vi "Dictionary New__ogtk.vi"(8 "error in (no error)":errorcluster, 10 "Data in":T2) -> (0 "error out":errorcluster, 3 "Object RefNum":T1)   [LabVIEW 2014]
doc: "Initializes the GOOP object"
uses:
  <userlib>/_OpenG.lib/dictionary/dictionary.llb/Dictionary Data__ogtk.ctl
  <userlib>/_OpenG.lib/dictionary/dictionary.llb/Dictionary Object RefNum__ogtk.ctl
  <userlib>/_OpenG.lib/dictionary/dictionary.llb/Dictionary Object RefNum - Enum__ogtk.ctl
panel:
  # "OpenGOOP New.vi\n\nInitializes the GOOP object\n\nPlease visit http://www.OpenG.org to learn about the\nOpen Source LabVIEW software movement.\n\nNOTICE -- YOU MUST LEAVE THIS NOTICE IN PLACE.  PER THE TERMS OF THE LICENSE BELOW, YOU MAY SUBLICENSE THIS SOFTWARE \nIN ANY WAY THAT DOES NOT CONFLICT WITH THIS LICENSE.\n\n### BSD License (http://www.opensource.org/licenses/bsd-license.php) Begin ###\n \nCopyright (c) 2003, Jim Kring <jim@jimkring.com>\n\nAll rights reserved.\n\nRedistribution and use in source and binary forms, with or without modification, are permitted provided that the following conditions are met:\n\n    * Redistributions of source code must retain the above copyright notice, this list of conditions and the following disclaimer.\n    * Redistributions in binary form must reproduce the above copyright notice, this list of conditions and the following disclaimer in the \n       documentation and/or other materials provided with the distribution.\n    * Neither the name of SciWare, James Kring, Inc., nor the names of its contributors may be used to endorse or promote products derived \n       from this software without specific prior written permission.\n\nTHIS SOFTWARE IS PROVIDED BY THE COPYRIGHT HOLDERS AND CONTRIBUTORS \"AS IS\" AND ANY EXPRESS OR IMPLIED WARRANTIES, \nINCLUDING, BUT NOT LIMITED TO, THE IMPLIED WARRANTIES OF MERCHANTABILITY AND FITNESS FOR A PARTICULAR PURPOSE ARE \nDISCLAIMED. IN NO EVENT SHALL THE COPYRIGHT OWNER OR CONTRIBUTORS BE LIABLE FOR ANY DIRECT, INDIRECT, INCIDENTAL,\n SPECIAL, EXEMPLARY, OR CONSEQUENTIAL DAMAGES (INCLUDING, BUT NOT LIMITED TO, PROCUREMENT OF SUBSTITUTE GOODS OR \nSERVICES; LOSS OF USE, DATA, OR PROFITS; OR BUSINESS INTERRUPTION) HOWEVER CAUSED AND ON ANY THEORY OF LIABILITY, \nWHETHER IN CONTRACT, STRICT LIABILITY, OR TORT (INCLUDING NEGLIGENCE OR OTHERWISE) ARISING IN ANY WAY OUT OF THE USE \nOF THIS SOFTWARE, EVEN IF ADVISED OF THE POSSIBILITY OF SUCH DAMAGE.\n\n### BSD License End ###"
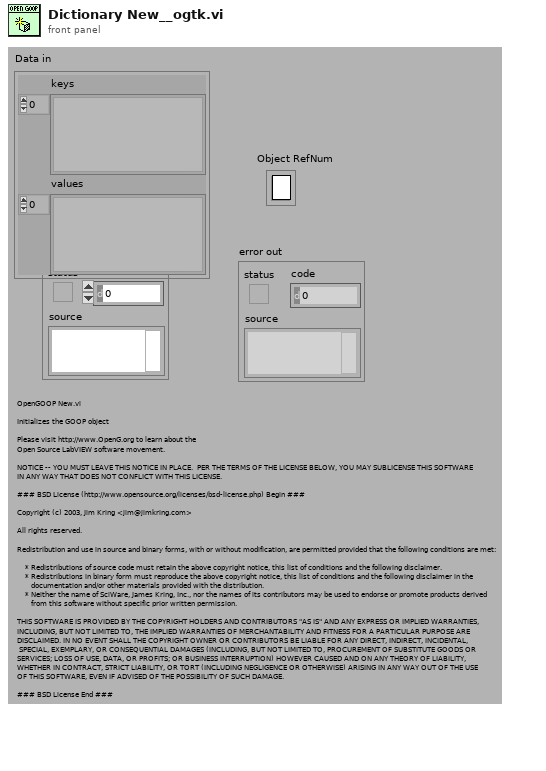
[diagram p1: front panel]
types:
  T1 = typedef "Dictionary Object RefNum__ogtk.ctl" = refnum<k1>
  T2 = typedef "Dictionary Data__ogtk.ctl" = cluster{"keys":variant[], "values":variant[]}
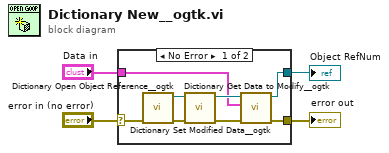
[diagram p0: block diagram]
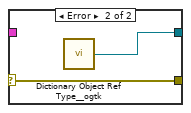
[diagram p2: hidden frame]
diagram:
  n1 = case shown="No Error" "error in (no error)" {
    selector: "error in (no error)" -> [w5 w14]
    tunnel: [w11 w14] -> w4
    tunnel: "Data in" -> [w8 _]
    tunnel: [w10 w13] -> w1
    frame No Error {
      n2 = call <userlib>:"Dictionary Open Object Reference__ogtk.vi"("error in (no error)"=w5) -> ("error out"=w7:errorcluster, "Object RefNum"=w6:T1)  [unwired: 9 in]
      n3 = call <userlib>:"Dictionary Get Data to Modify__ogtk.vi"("error in (no error)"=w7, "Object RefNum"=w6) -> ("error out"=w12:errorcluster, "Dup Object RefNum"=w9:T1)  [unwired: 6 in, 2 out]
      n4 = call <userlib>:"Dictionary Set Modified Data__ogtk.vi"("error in (no error)"=w12, "Data in"=w8, "Object RefNum"=w9) -> ("error out"=w11:errorcluster, "dup Object RefNum"=w10:T1)  [unwired: 7 in]
    }
    frame Error {
      n5 = call <userlib>:"Dictionary Object Ref Type__ogtk.vi"() -> ("Object RefNum Type"=w13:T1)  [unwired: 5 in]
    }
  }
  "error out" <- w4
  "Object RefNum" <- w1
